vi "Global MAP.vi"(5 "Start point":dbl[](array[numeric]), 7 "Start Front point":dbl[](array[numeric]), 8 "Y point":dbl[](array[numeric]), 10 "X point":dbl[](array[numeric])) -> (2 "ODM Global Lidar":cluster{dbl[], dbl[]}[](graph))   [LabVIEW 2018]
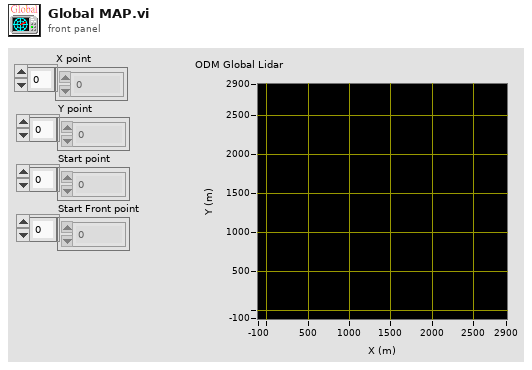
[diagram p1: front panel]
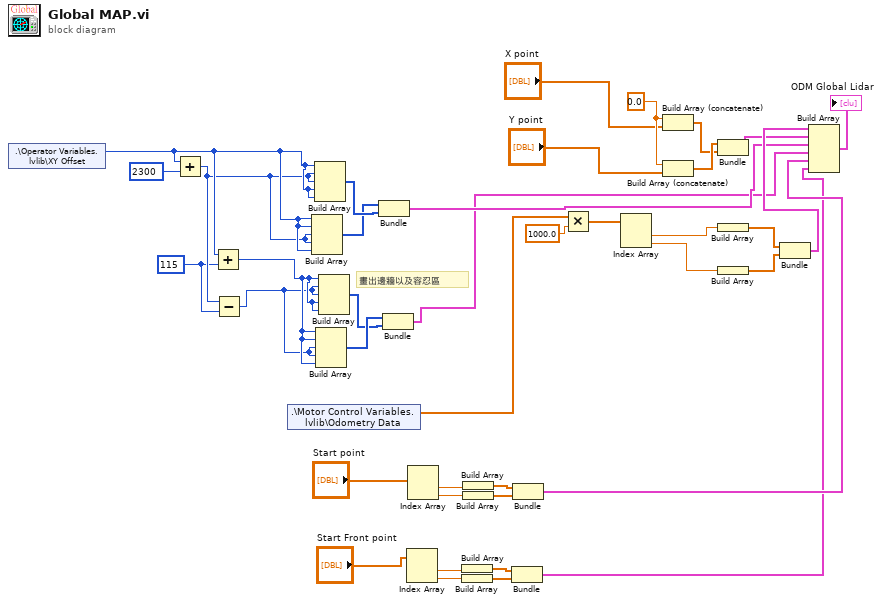
[diagram p0: block diagram]
diagram:
  w15 = i16 115 ("y")
  w35 = 0.0 ("element")
  # "畫出邊牆以及容忍區"
  n1 = shared-variable ".\\Operator Variables.lvlib\\XY Offset"() -> (w17:i16)  [unwired: 1 in, 1 out]
  n2 = Add(x=w17, y=i16 2300) -> (x+y=w16:i16)
  n3 = Add(x=w17, y=w15) -> (x+y=w14:i16)
  n4 = Subtract(x=w16, y=w15) -> (x-y=w13:i16)
  n5 = shared-variable ".\\Motor Control Variables.lvlib\\Odometry Data"() -> (w22:dbl[])  [unwired: 1 in, 1 out]
  n6 = Build Array(w17, w17, w16, w16, w17) -> (w27:i16[])
  n7 = Build Array(w17, w16, w16, w17, w17) -> (w28:i16[])
  n8 = Build Array(w14, w14, w13, w13, w14) -> (w26:i16[])
  n9 = Build Array(w14, w13, w13, w14, w14) -> (w25:i16[])
  n10 = Bundle(w27, w28) -> (w24:cluster{i16[], i16[]})  [unwired: 1 in]
  n11 = Bundle(w26, w25) -> (w23:cluster{i16[], i16[]})  [unwired: 1 in]
  n12 = Index Array(array="Start Front point") -> (element #1=w5:dbl, element #2=w6:dbl)  [unwired: 2 in]
  n13 = Index Array(array="Start point") -> (element #1=w9:dbl, element #2=w8:dbl)  [unwired: 2 in]
  n14 = Build Array(w5) -> (w4:dbl[])
  n15 = Build Array(w6) -> (w3:dbl[])
  n16 = Build Array(w9) -> (w10:dbl[])
  n17 = Build Array(w8) -> (w11:dbl[])
  n18 = Bundle(w4, w3) -> (w1:cluster{dbl[], dbl[]})  [unwired: 1 in]
  n19 = Bundle(w10, w11) -> (w7:cluster{dbl[], dbl[]})  [unwired: 1 in]
  n20 = Multiply(x=w22, y=1000.0 ("element")) -> (x*y=w21:dbl[])
  n21 = Index Array(array=w21) -> (element #1=w39:dbl, element #2=w38:dbl)  [unwired: 2 in]
  n22 = Build Array (concatenate)(w35, "X point") -> (w30:dbl[])
  n23 = Build Array (concatenate)(w35, "Y point") -> (w31:dbl[])
  n24 = Bundle(w31, w30) -> (w34:cluster{dbl[], dbl[]})  [unwired: 1 in]
  n25 = Build Array(w39) -> (w33:dbl[])
  n26 = Build Array(w38) -> (w32:dbl[])
  n27 = Bundle(w33, w32) -> (w37:cluster{dbl[], dbl[]})  [unwired: 1 in]
  n28 = Build Array(w37, w34, w24, w23, w7, w1) -> (→"ODM Global Lidar":cluster{dbl[], dbl[]}[])
